vi "난수발생(4-3).vi"() -> ()   [LabVIEW 2014]
panel:
  in  "경로":path
  in  "가운데로":bool
  in  "메뉴바/도구바":bool
  in  "정지":bool
  in  "난수 발생":bool
  out "웨이브폼 차트":dbl(graph)
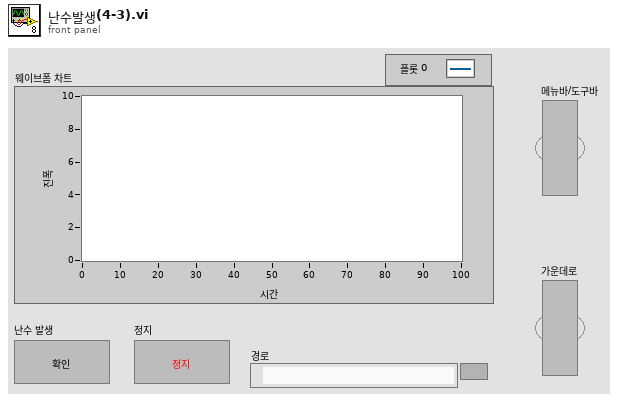
[diagram p1: front panel]
types:
  T1 = enum16{"Always On", "Always Off", "Off While Running"}
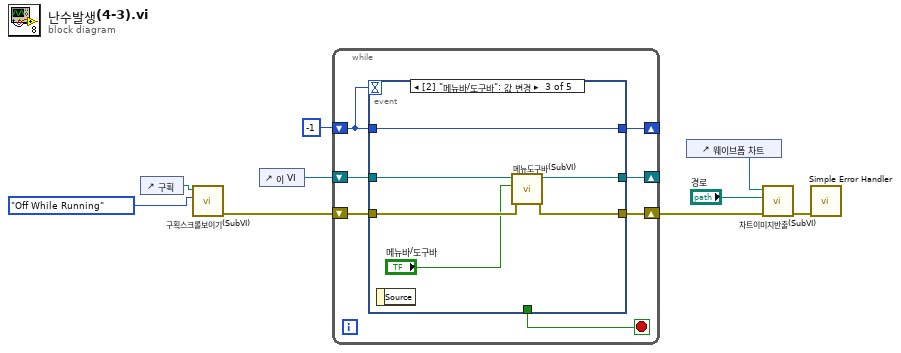
[diagram p0: block diagram]
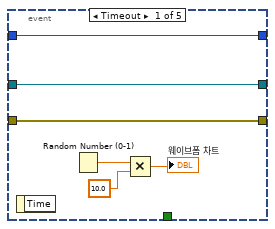
[diagram p2: hidden frame]
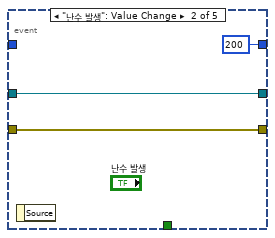
[diagram p3: hidden frame]
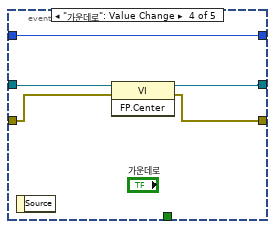
[diagram p4: hidden frame]
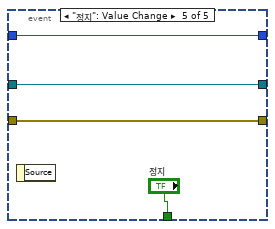
[diagram p5: hidden frame]
diagram:
  n1 = control-ref of="구획"() -> (w2:refnum<vi>)
  n2 = call "구획스크롤보이기(SubVI).vi"("수직 스크롤 막대 보이기"=T1."Off While Running", "Pane 입력"=w2) -> ("에러 출력"=w6:errorcluster)  [unwired: 9 in]
  n3 = control-ref of="이 VI"() -> (w8:refnum<vi>)
  n4 = while {
    shift-right: [w15] -> _
    shift-left: -1 -> [w16]
    shift-right: [w11] -> _
    shift-left: w8 -> [w13]
    shift-right: [w10] -> w5
    shift-left: w6 -> [w12]
    stop <- w14 stop-if-true
    n5 = event shown="[2] \"메뉴바/도구바\": 값 변경" {
      selector: _ -> [_ _ _ _ _]
      dyn-events: _ -> [_ _ _ _ _]
      timeout: w16 -> [_ _ _ _ _]
      tunnel: [w22 200 w31 w36 w39] -> w15
      tunnel: w16 -> [w22 _ w31 w36 w39]
      tunnel: [_ _ _ _ "정지"] -> w14
      tunnel: w13 -> [w18 w25 w29 w35 w38]
      tunnel: w12 -> [w17 w24 w28 w33 w37]
      tunnel: [w18 w25 w30 w34 w38] -> w11
      tunnel: [w17 w24 w27 w32 w37] -> w10
      event Timeout {
        n6 = event-data() -> ()  [unwired: 1 in, 1 out]
        n7 = Random Number (0-1)() -> (number: 0 to 1=w20:dbl)
        n8 = Multiply(x=w20, y=10.0) -> (x*y=→"웨이브폼 차트":dbl)
      }
      event "난수 발생": Value Change {
        n9 = event-data() -> ()  [unwired: 1 in, 1 out]
      }
      event "메뉴바/도구바": Value Change {
        n10 = event-data() -> ()  [unwired: 1 in, 1 out]
        n11 = call "메뉴도구바(SubVI).vi"("에러 입력(에러 없음)"=w28, "메뉴바/도구바"="메뉴바/도구바", "VI 입력"=w29) -> ("에러 출력"=w27:errorcluster, "VI 출력"=w30:refnum<vi>)  [unwired: 7 in]
      }
      event "가운데로": Value Change {
        n12 = event-data() -> ()  [unwired: 1 in, 1 out]
        n13 = invoke class="VI" method="FP.Center"(reference=w35, error in=w33) -> (reference out=w34:refnum<vi>, error out=w32:errorcluster)  [unwired: 1 in, 1 out]
      }
      event "정지": Value Change {
        n14 = event-data() -> ()  [unwired: 1 in, 1 out]
      }
    }
  }
  n15 = control-ref of="웨이브폼 차트"() -> (w1:refnum<vi>)
  n16 = call "차트이미지반출(SubVI).vi"("에러 입력(에러 없음)"=w5, "경로"="경로", "WaveformChart 입력"=w1) -> ("에러 출력"=w3:errorcluster)  [unwired: 8 in]
  n17 = call <vilib>:"Simple Error Handler.vi"("error in (no error)"=w3) -> ()  [unwired: 4 in, 5 out]
